vi "FPGA Main.vi"() -> ()   [LabVIEW 2012]
uses:
  Type/_RW Status.ctl
  Type/_LED States.ctl
  Type/_FPGA States.ctl
  Type/_FPGA DC Lines.ctl
  <vilib>/Platform/TimedLoop/XDataNode/timing_clust.ctl
  <vilib>/Platform/TimedLoop/XDataNode/nitl_modes.ctl
  <vilib>/Platform/TimedLoop/XDataNode/wakeup.ctl
  <vilib>/rvi/Emulation/niFpgaSctlEmulationGetInTimedLoop.vi
  <vilib>/rvi/DataTransferAndStorage/Container/Common/niFpgaContainerGetUniqueNameForEmu.vi
  <vilib>/rvi/Memory/Memory_Emulation/niFpgaMemoryEmulationCacheClearOnFirstRun.vi
  <vilib>/rvi/Memory/Memory_Emulation/nirvimemoryEmulationManagerCache_MakeExclusive.vi
  <vilib>/rvi/Memory/Memory_Emulation/niFpgaMemoryEmulationValidateCache.vi
  <vilib>/rvi/Memory/Memory_Emulation/nirvimemoryEmulationManagerCache_ReleaseExclusive.vi
  <vilib>/rvi/Memory/Memory_Emulation/nirvimemoryEmulationManagerCache_InsertValue.vi
  <vilib>/Utility/error.llb/Clear Errors.vi
  <vilib>/rvi/Memory/Memory_Emulation/nirvimemoryEmulationManagerCache_GetValue.vi
  <vilib>/rvi/Emulation/niFpgaSctlEmulationGlobalWrite.vi
  <vilib>/rvi/Memory/Memory_Emulation/nirvimemoryEmulationManagerCache_SetValue.vi
  <vilib>/rvi/Emulation/niFpgaSctlEmulationResourceMgr.vi
  <vilib>/rvi/eio/common/nirviEmuTemplateMethod_errors.vi
  <vilib>/rvi/Emulation/niFpgaSctlEmulationRegisterWithScheduler.vi
  <vilib>/rvi/Emulation/niFpgaSctlEmulationScheduler.vi
  Instance           1 17Saved   FPGA Main .vi
  Instance           2 17Saved   FPGA Main .vi
  <vilib>/rvi/interface/RandomDataEmulation/nirviRandomDataFPGAFIFO.vi
  <vilib>/rvi/interface/RandomDataEmulation/niFpgaRandomDataHandleErrors.vi
  <vilib>/rvi/DataTransferAndStorage/Container/XNode/niFpgaContainer.xnode
  <vilib>/rvi/Memory/Memory_Emulation/nirvimemoryEmulation.vi
  <vilib>/eio/EIONode/EIONode.xnode
  <vilib>/Platform/TimedLoop/XDataNode/XDataNode.xnode
  <vilib>/rvi/interface/RandomDataEmulation/nirviRandomDataFpgaReadWriteTemplate.vi
  <vilib>/Platform/TimedLoop/XDataNode/XDNodeRunTimeDep.lvlib
panel:
  in  "FilaB":bool
  in  "FilaC":bool
  in  "Send Serial":bool
  in  "Repeat":bool
  in  "LED States":T1
  in  "Update":bool
  out "Version":u32=900130925
  in  "R/W Status":T2
  in  "Start":bool
  out "Running":bool
  in  "Address":u16
  in  "Data":u32
  in  "Read/Write":bool
  # "Memory Map Access"
  # "Run Cycle Control"
  # "VG Filament Control"
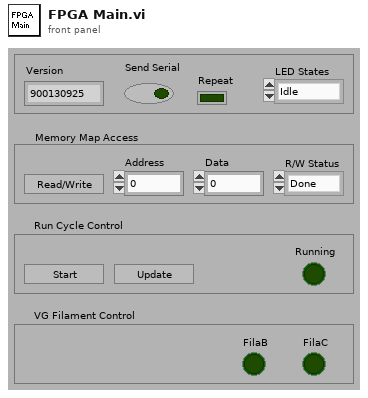
[diagram p1: front panel]
types:
  T1 = typedef "_LED States.ctl" = enum8{"Idle", "Solid B", "Solid R", "Solid P", "Off B", "Off R", "Off P", "Off BRP", "Off RP", "Flash R&P", "Flash P"}
  T2 = typedef "_RW Status.ctl" = enum8{"Done", "Do Read", "Do Write", "Set Latch1", "Set Latch2", "Set Latch3", "Set Latch4", "RP ON", "EL ON", "Serial Send", "Set LC Out", "Get LC In", "Read VAC", "Table Test", "Get Interlock", "Do Read2", "Do Write2"}
  T3 = typedef "_FPGA States.ctl" = enum8{"Wait", "Single", "Dual", "DoCycles", "RampParam", "ReadADC", "SetOscil", "SetPIC", "EleOn", "Stop"}
  T4 = typedef "XDNodeRunTimeDep.lvlib/timing_clust.ctl" = cluster{"Expected End [f-1]":u64, "Actual End [f-1]":u64, "Finished Late? [f-1]":bool, "Expected End [i-1]":u64, "Actual End [i-1]":u64, "Finished Late? [i-1]":bool, "Expected Start [i]":u64, "Actual Start [i]":u64, "Expected Start [f]":u64, "Actual Start [f]":u64, "Source Name":string, "Structure Name":string, "Period":i64, "Deadline":i64, "Offset":i64, "Start":i64, "Priority":i32, "Timeout":i32, "Mode":T5, "Wakeup Reason":T6, "Error":errorcluster, "Source Type":string, "Secondary Source Type":string, "Global End Time":u64, "Global Start Time":u64, "Frame Duration":u64, "Iteration Duration":u64, "Assigned CPU":i32, "I/O Scan Engine Mode":u32}
  T5 = typedef "XDNodeRunTimeDep.lvlib/nitl_modes.ctl" = enum32{"No Change", "Process missed periods, maintain original phase", "Discard missed periods, maintain original phase", "Process missed periods, ignore original phase", "Discard missed periods, ignore original phase"}
  T6 = typedef "XDNodeRunTimeDep.lvlib/wakeup.ctl" = enum32{"Normal", "Aborted", "Asynchronous wakeup", "Timing source error", "Timed loop error", "Timeout"}
  T7 = typedef "_FPGA DC Lines.ctl" = enum16{"Q1 POL", "Q3 POL", "Q1 DC EN", "Q3 DC EN", "COR POL", "CUR POL", "S1 POL", "S2 POL", "CEM POL"}
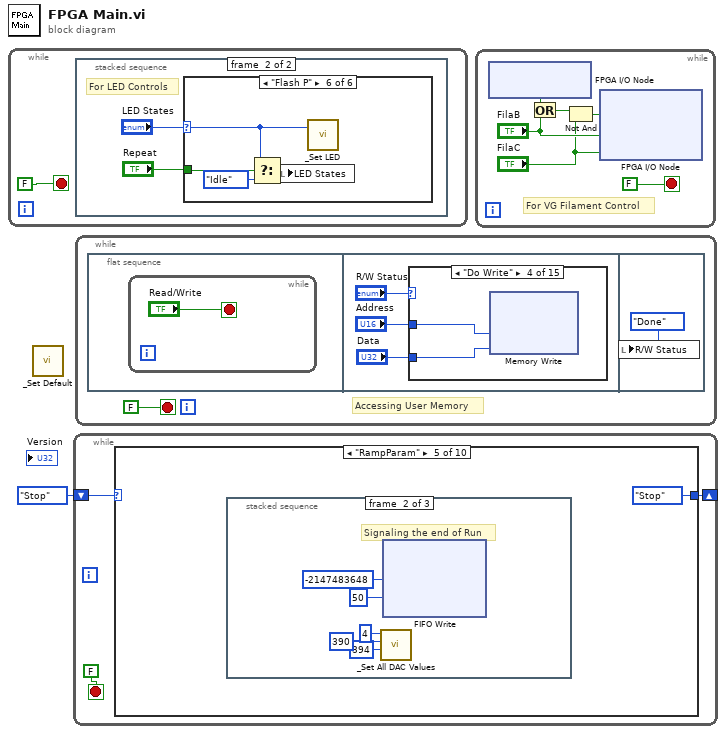
[diagram p0: block diagram]
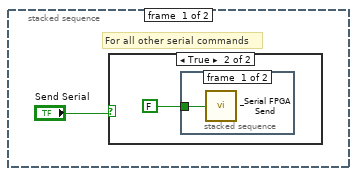
[diagram p2: hidden frame]
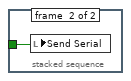
[diagram p4: hidden frame]
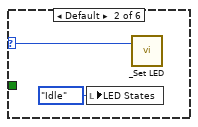
[diagram p6: hidden frame]
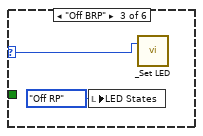
[diagram p7: hidden frame]
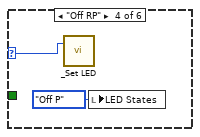
[diagram p8: hidden frame]
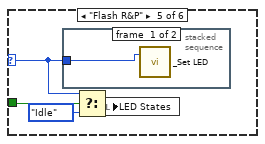
[diagram p9: hidden frame]
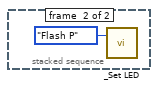
[diagram p10: hidden frame]
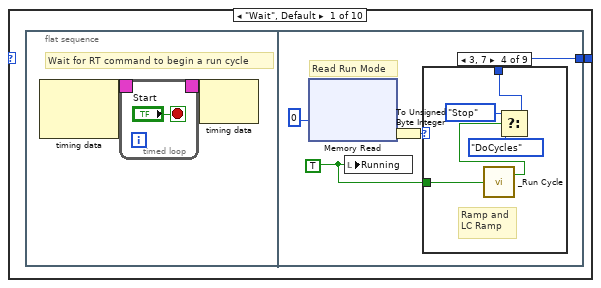
[diagram p11: hidden frame]
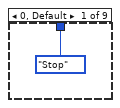
[diagram p12: hidden frame]
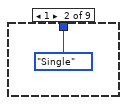
[diagram p13: hidden frame]
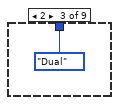
[diagram p14: hidden frame]
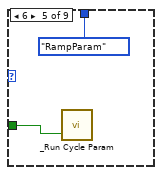
[diagram p15: hidden frame]
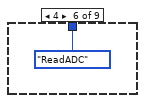
[diagram p16: hidden frame]
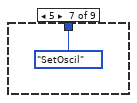
[diagram p17: hidden frame]
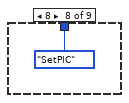
[diagram p18: hidden frame]
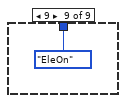
[diagram p19: hidden frame]
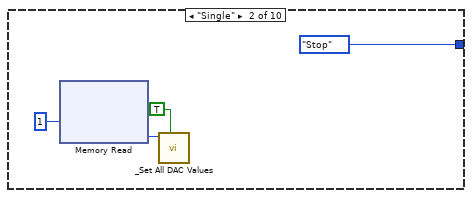
[diagram p20: hidden frame]
diagram:
  n1 = while {
    stop <- FALSE stop-if-true
    n2 = stacked-sequence {
      frame #0 {
        # "For all other serial commands"
        n3 = case shown="True" "Send Serial" {
          frame False {
          }
          frame True {
            n4 = stacked-sequence {
              tunnel: FALSE ("LED Control (T)") -> [w5 w6]
              frame #0 {
                n5 = call "_Serial FPGA Send.vi"("LED Control (T)"=w5) -> ()
              }
              frame #1 {
                n6 = local write "Send Serial"(w6) -> ()
              }
            }
          }
        }
      }
      frame #1 {
        # "For LED Controls"
        n7 = case shown="\"Flash P\"" "LED States" {
          selector: "LED States" -> [_ w9 w11 w13 w15 w21]
          tunnel: "Repeat" -> [_ _ _ _ w18 w24]
          frame "Idle" {
          }
          frame Default {
            n8 = local write "LED States"(_LED_States."Idle" ("LED States")) -> ()
            n9 = call "_Set LED.vi"("LED States"=w9) -> ()  [unwired: 3 out]
          }
          frame "Off BRP" {
            n10 = local write "LED States"(_LED_States."Off RP" ("LED States")) -> ()
            n11 = call "_Set LED.vi"("LED States"=w11) -> ()  [unwired: 3 out]
          }
          frame "Off RP" {
            n12 = call "_Set LED.vi"("LED States"=w13) -> ()  [unwired: 3 out]
            n13 = local write "LED States"(_LED_States."Off P" ("LED States")) -> ()
          }
          frame "Flash R&P" {
            n14 = stacked-sequence {
              tunnel: w15 -> [w19 _]
              frame #0 {
                n15 = call "_Set LED.vi"("LED States"=w19) -> ()  [unwired: 3 out]
              }
              frame #1 {
                n16 = call "_Set LED.vi"("LED States"=_LED_States."Flash P") -> ()  [unwired: 3 out]
              }
            }
            n17 = Select(t=w15, s=w18, f=_LED_States."Idle") -> (s? t:f=w17:T1)
            n18 = local write "LED States"(w17) -> ()
          }
          frame "Flash P" {
            n19 = Select(t=w21, s=w24, f=_LED_States."Idle") -> (s? t:f=w23:T1)
            n20 = local write "LED States"(w23) -> ()
            n21 = call "_Set LED.vi"("LED States"=w21) -> ()  [unwired: 3 out]
          }
        }
      }
    }
  }
  n22 = call "_Set Default.vi"() -> ()  [unwired: 6 out]
  n23 = while {
    shift-right: [w26] -> _
    shift-left: _FPGA_States."Stop" ("FPGA States") -> [w27]
    stop <- FALSE stop-if-true
    n24 = case shown="\"RampParam\"" w27 {
      tunnel: [w28 _FPGA_States."Stop" ("FPGA States") _FPGA_States."Stop" ("FPGA States") _FPGA_States."Stop" ("FPGA States") _FPGA_States."Stop" ("FPGA States") _FPGA_States."Stop" ("FPGA States") _FPGA_States."Stop" ("FPGA States") _FPGA_States."Stop" ("FPGA States") _FPGA_States."Stop" ("FPGA States") _FPGA_States."Wait" ("FPGA States")] -> w26
      frame "Wait", Default {
        n25 = flat-sequence {
          tunnel: [w40] -> w28
          frame #0 {
            # "Wait for RT command to begin a run cycle"
            n26 = node-c288() -> (w29:T4)  [unwired: 2 out]
            n27 = timed-loop {
              timing-out: [_] -> w30
              timing: w29 -> [_]
              stop <- "Start" stop-if-true
            }
            n28 = node-c288(w30) -> ()  [unwired: 1 out]
          }
          frame #1 {
            w36 = TRUE ("Running")
            # "Read Run Mode"
            n29 = xnode ("Memory Read")("Address"=u8 0) -> ("Data"=w39:u32)  [unwired: 1 in, 1 out]
            n30 = local write "Running"(w36) -> ()
            n31 = To Unsigned Byte Integer(number=w39) -> (unsigned 8bit integer=w37:u8)
            n32 = case shown="3, 7" w37 {
              tunnel: [_FPGA_States."Stop" ("FPGA States") _FPGA_States."Single" ("FPGA States") _FPGA_States."Dual" ("FPGA States") w45 _FPGA_States."RampParam" ("FPGA States") _FPGA_States."ReadADC" ("FPGA States") _FPGA_States."SetOscil" ("FPGA States") _FPGA_States."SetPIC" ("FPGA States") _FPGA_States."EleOn" ("FPGA States")] -> w40
              tunnel: w36 -> [_ _ _ w44 w49 _ _ _ _]
              frame 0, Default {
              }
              frame 1 {
              }
              frame 2 {
              }
              frame 3, 7 {
                # "Ramp and\nLC Ramp"
                n33 = call "_Run Cycle.vi"("Init (F)"=w44) -> ("Finish Run?"=w48:bool)  [unwired: 2 in, 1 out]
                n34 = Select(t=_FPGA_States."Stop" ("FPGA States"), s=w48, f=_FPGA_States."DoCycles" ("FPGA States")) -> (s? t:f=w45:T3)
              }
              frame 6 {
                n35 = call "_Run Cycle Param.vi"("Init (F)"=w49) -> ()  [unwired: 2 out]
              }
              frame 4 {
              }
              frame 5 {
              }
              frame 8 {
              }
              frame 9 {
              }
            }
          }
        }
      }
      frame "Single" {
        n36 = xnode ("Memory Read")("Address"=u8 1) -> ("Data"=w56:u32)  [unwired: 1 in, 1 out]
        n37 = call "_Set All DAC Values.vi"("Record Values (F)"=TRUE, "# of Active Channels"=w56) -> ()  [unwired: 7 in]
      }
      frame "Dual" {
        w61 = u8 1 ("Address")
        # "Run until a Cancel command is received"
        n38 = Increment(x=w61) -> (x+1=w59:u8)
        n39 = Increment(x=w59) -> (x+1=w60:u8)
        n40 = xnode ("Memory Read")("Address"=w61) -> ("Data"=w64:u32)  [unwired: 1 in, 1 out]
        n41 = xnode ("Memory Read")("Address"=w59) -> ("Data"=w63:u32)  [unwired: 1 in, 1 out]
        n42 = xnode ("Memory Read")("Address"=w60) -> ("Data"=w62:u32)  [unwired: 1 in, 1 out]
        n43 = while {
          tunnel: w63 -> [w72]
          tunnel: w62 -> [w71]
          tunnel: w64 -> [w70]
          stop <- w67 stop-if-true
          w66 = u8 0 ("Address")
          # "Read High Level Time (uS)"
          # "Read Low Level Time (uS)"
          n44 = xnode ("Memory Read")("Address"=w66) -> ("Data"=w69:u32)  [unwired: 1 in, 1 out]
          n45 = To Unsigned Byte Integer(number=w69) -> (unsigned 8bit integer=w68:u8)
          n46 = stacked-sequence {
            tunnel: w72 -> [w75 _]
            tunnel: w71 -> [_ w78]
            tunnel: w70 -> [w74 w77]
            frame #0 {
              n47 = call "Wait"("Count(uSec)"=w75) -> ()  [unwired: 1 out]
              n48 = call "_Set All DAC Values.vi"("Record Values (F)"=TRUE, "# of Active Channels"=w74) -> ()  [unwired: 7 in]
            }
            frame #1 {
              w79 = u16 130  # Low Value Offset
              n49 = call "Wait1"("Count(uSec)"=w78) -> ()  [unwired: 1 out]
              n50 = call "_Set All DAC Values.vi"("Record Values (F)"=TRUE, "DAC Value Offset (70)"=w79, "# of Active Channels"=w77) -> ()  [unwired: 6 in]
            }
          }
          n51 = Equal?(x=w68, y=w66) -> (x = y?=w67:bool)
        }
      }
      frame "DoCycles" {
        n52 = stacked-sequence {
          frame #0 {
            n53 = while {
              tunnel: [w85] -> w81
              i -> [w85]
              stop <- w83 stop-if-true
              n54 = call "_Run Cycle.vi"("Update"="Update") -> ("Finish Run?"=w83:bool)  [unwired: 1 in, 2 out]
            }
            n55 = xnode ("Memory Write")("Address"=u8 7, "Data"=w81) -> ()  [unwired: 1 in, 1 out]
          }
          frame #1 {
            # "Signaling the end of Run"
            n56 = xnode ("FIFO Write")("Element"=-2147483648, "Timeout"=u8 50 ("Timeout (-1 for no timeout)")) -> ()  [unwired: 1 in, 2 out]
            n57 = call "_Set All DAC Values.vi"("DAC Value Offset (70)"=u16 394, "Channel ID Offset (10)"=u16 390, "# of Active Channels"=u16 4) -> ()  [unwired: 6 in]
          }
          frame #2 {
            # "Turn off LC Stop"
            n58 = call "_Update LC Out.vi"("LC Stop"=FALSE, "LC Hold"=TRUE) -> ()  [unwired: 6 out]
          }
        }
      }
      frame "RampParam" {
        n59 = stacked-sequence {
          frame #0 {
            n60 = while {
              tunnel: [w100] -> w94
              i -> [w100]
              stop <- w101 stop-if-true
              w97 = u8 0 ("Address")
              n61 = xnode ("Memory Read")("Address"=w97) -> ("Data"=w99:u32)  [unwired: 1 in, 1 out]
              n62 = call "_Run Cycle Param.vi"() -> ("Finish Run?"=w102:bool)  [unwired: 1 in, 1 out]
              n63 = To Unsigned Byte Integer(number=w99) -> (unsigned 8bit integer=w98:u8)
              n64 = Equal?(x=w98, y=w97) -> (x = y?=w96:bool)
              n65 = Or(x=w102, y=w96) -> (x .or. y?=w101:bool)
            }
            n66 = xnode ("Memory Write")("Address"=u8 7, "Data"=w94) -> ()  [unwired: 1 in, 1 out]
          }
          frame #1 {
            # "Signaling the end of Run"
            n67 = call "_Set All DAC Values.vi"("DAC Value Offset (70)"=u16 394, "Channel ID Offset (10)"=u16 390, "# of Active Channels"=u16 4) -> ()  [unwired: 6 in]
            n68 = xnode ("FIFO Write")("Element"=-2147483648, "Timeout"=u8 50 ("Timeout (-1 for no timeout)")) -> ()  [unwired: 1 in, 2 out]
          }
          frame #2 {
            # "Turn off LC Stop"
            n69 = call "_Update LC Out.vi"("LC Stop"=FALSE, "LC Hold"=TRUE) -> ()  [unwired: 6 out]
          }
        }
      }
      frame "ReadADC" {
        n70 = for {
          N: u8 128 -> [_]
          i -> [w112]
          # "Read all ADC Values"
          n71 = call "_Read ADC.vi"("Channel #"=w112) -> ()  [unwired: 1 out]
        }
      }
      frame "SetOscil" {
        n72 = call "_Set Oscillator.vi"() -> ()  [unwired: 2 out]
      }
      frame "SetPIC" {
        w117 = u8 7 ("Address")
        n73 = Increment(x=w117) -> (x+1=w116:u8)
        n74 = xnode ("Memory Read")("Address"=w117) -> ("Data"=w115:u32)  [unwired: 1 in, 1 out]
        n75 = xnode ("Memory Read")("Address"=w116) -> ("Data"=w114:u32)  [unwired: 1 in, 1 out]
        n76 = call "_Set 1 DAC Value.vi"("DAC"=w114, "Ch#"=w115) -> ()  [unwired: 2 out]
      }
      frame "EleOn" {
        n77 = call "_Electronic On.vi"() -> ()  [unwired: 1 out]
      }
      frame "Stop" {
        n78 = flat-sequence {
          frame #0 {
            n79 = call "_Chip Select.vi"() -> ()  [unwired: 1 in, 7 out]
          }
          frame #1 {
            n80 = call "_Update Serial DAC.vi"() -> ()  [unwired: 4 in, 4 out]
          }
          frame #2 {
            "Running" <- FALSE
          }
        }
      }
    }
  }
  n81 = while {
    stop <- FALSE stop-if-true
    # "Accessing User Memory"
    n82 = flat-sequence {
      frame #0 {
        n83 = while {
          stop <- "Read/Write" stop-if-true
        }
      }
      frame #1 {
        n84 = case shown="\"Do Write\"" "R/W Status" {
          tunnel: "Address" -> [_ w128 w130 w132 w134 w135 w137 w139 w141 w143 w149 _ _ _ _]
          tunnel: "Data" -> [_ _ _ w131 w133 _ _ _ _ _ _ _ _ _ _]
          frame "Done", Default {
          }
          frame "Do Read" {
            n85 = xnode ("Memory Read")("Address"=w128) -> ("Data"=w127:u32)  [unwired: 1 in, 1 out]
            n86 = local write "Data"(w127) -> ()
          }
          frame "Do Read2" {
            n87 = xnode ("Memory Read")("Address"=w130) -> ("Data"=w129:u32)  [unwired: 1 in, 1 out]
            n88 = local write "Data"(w129) -> ()
          }
          frame "Do Write" {
            n89 = xnode ("Memory Write")("Address"=w132, "Data"=w131) -> ()  [unwired: 1 in, 1 out]
          }
          frame "Do Write2" {
            n90 = xnode ("Memory Write")("Address"=w134, "Data"=w133) -> ()  [unwired: 1 in, 1 out]
          }
          frame "Set Latch1" {
            n91 = call "_Set DC Line.vi"("States"=w135, "DC Line"=_FPGA_DC_Lines."Q1 POL") -> ()  [unwired: 2 out]
          }
          frame "Set Latch2" {
            n92 = call "_Set DC Line.vi"("States"=w137, "DC Line"=_FPGA_DC_Lines."COR POL") -> ()  [unwired: 2 out]
          }
          frame "Set Latch3" {
            n93 = call "_Set DC Line.vi"("States"=w139, "DC Line"=_FPGA_DC_Lines."S1 POL") -> ()  [unwired: 2 out]
          }
          frame "Set Latch4" {
            n94 = call "_Set DC Line.vi"("States"=w141, "DC Line"=_FPGA_DC_Lines."CEM POL") -> ()  [unwired: 2 out]
          }
          frame "RP ON" {
            n95 = Greater Than 0?(x=w143) -> (x > 0?=w144:bool)
            n96 = xnode "FPGA I/O Node"("Port1/DIO9"=w144) -> ()  [unwired: 1 in, 1 out]
          }
          frame "Set LC Out" {
            n97 = Number To Boolean Array(number=w149) -> (Boolean array=w150:bool[])
            n98 = Index Array(array=w150) -> (element #1=w148:bool, element #2=w147:bool, element #3=w146:bool, element #4=w145:bool)  [unwired: 4 in]
            n99 = xnode "FPGA I/O Node"("Port5/DIO5"=w148, "Port5/DIO6"=w147, "Port5/DIO8"=w146, "Port6/DIO3"=w145) -> ()  [unwired: 4 in, 4 out]
          }
          frame "Get LC In" {
            # "LC2-I1"
            # "LC1-I1"
            n100 = xnode "FPGA I/O Node"() -> ("Port5/DIO7"=w155:bool, "Port6/DIO0"=w154:bool)  [unwired: 2 in, 2 out]
            n101 = Boolean To (0,1)(Boolean=w154) -> (0, 1=w152:i16)
            n102 = Boolean To (0,1)(Boolean=w155) -> (0, 1=w153:i16)
            n103 = Join Numbers(hi=w153, lo=w152) -> ((hi.lo)=w151:u32)
            n104 = local write "Data"(w151) -> ()
          }
          frame "Get Interlock" {
            # "Card cage door"
            n105 = xnode "FPGA I/O Node"() -> ("Port6/DIO7"=w157:bool)  [unwired: 1 in, 1 out]
            n106 = Boolean To (0,1)(Boolean=w157) -> (0, 1=w156:i16)
            n107 = local write "Data"(w156) -> ()
          }
          frame "Read VAC" {
            n108 = call "_Read VAC Gauge.vi"() -> ("DAC"=w158:u8)
            n109 = local write "Data"(w158) -> ()
          }
          frame "Table Test" {
            n110 = call "_Table Test.vi"() -> ()  [unwired: 1 out]
          }
        }
      }
      frame #2 {
        n111 = local write "R/W Status"(_RW_Status."Done" ("RW Status")) -> ()
      }
    }
  }
  n112 = while {
    stop <- FALSE stop-if-true
    # "For VG Filament Control"
    n113 = xnode "FPGA I/O Node"() -> ("Port2/DIO4"=w164:bool)  [unwired: 1 in, 1 out]
    n114 = Or(x=w164, y="FilaB") -> (x .or. y?=w163:bool)
    n115 = Not And(1:"FilaC", 2:w163) -> (0:w162:bool)
    n116 = xnode "FPGA I/O Node"("Port2/DIO7"=w162, "Port2/DIO5"="FilaB", "Port2/DIO6"="FilaC") -> ()  [unwired: 3 in, 3 out]
  }
